vi "Write Sweep Sequence Configuration.vi"(8 "error in (no error)":errorcluster, 10 "Configuration":T1 {"Duration" format="%#_6ps"}, 11 "Sweep Sequence in":refnum<class "Sweep.lvclass">) -> (0 "error out":errorcluster, 3 "Sweep Sequence out":refnum<class "Sweep.lvclass">)   [LabVIEW 2018, in "Sweep.lvclass"]
uses:
  Sweep.lvclass
  C:/github/LabActor/Template Module/Template Module.lvclass
  Sweep Sequence Configuration.ctl
  Template Module/Template Module.lvclass/Template Module.ctl
  Template Module/Write Configuration.vi
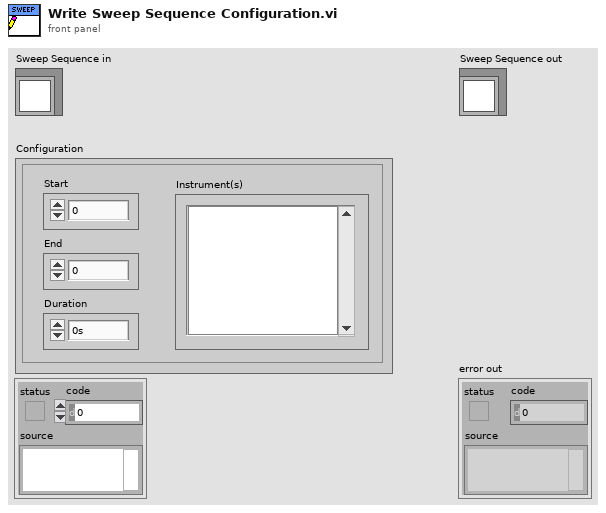
[diagram p1: front panel]
types:
  T1 = typedef "Sweep Sequence Configuration.ctl" = cluster{"Start":dbl, "End":dbl, "Duration":dbl, "Instrument(s)":i32}
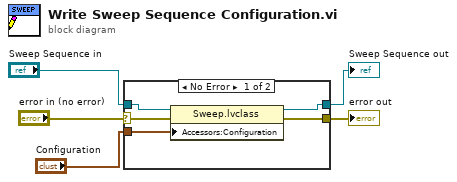
[diagram p0: block diagram]
diagram:
  n1 = case shown="No Error" "error in (no error)" {
    selector: "error in (no error)" -> [w10 w11]
    tunnel: [w9 w11] -> w4
    tunnel: [w7 w12] -> w2
    tunnel: "Sweep Sequence in" -> [w8 w12]
    tunnel: "Configuration" -> [w6 _]
    frame No Error {
      n2 = property class="Sweep.lvclass"(reference=w8, error in=w10, "Accessors:Configuration"=w6) -> (reference out=w7:refnum<class "Sweep.lvclass">, error out=w9:errorcluster)
    }
    frame Error {
    }
  }
  "error out" <- w4
  "Sweep Sequence out" <- w2
